vi "Update FLS Laser ID.vi"(8 "error in (no error)":errorcluster, 10 "DLS Laser ID (A,B,C or D)":enum16{"A", "B", "C", "D"}(ring), 11 "DLS Laser Actor in":refnum<class "FLS Laser Actor.lvclass">) -> (0 "error out":errorcluster, 3 "DLS Laser Actor out":refnum<class "FLS Laser Actor.lvclass">)   [LabVIEW 2018, in "FLS Laser Actor.lvlib" / "FLS Laser Actor.lvclass"]
uses:
  FLS Laser Actor.lvclass
  FLS Laser Actor.lvclass/FLS Laser Actor.ctl
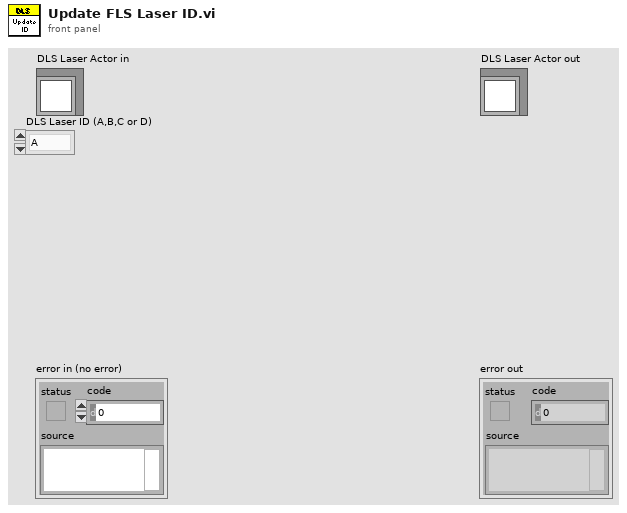
[diagram p1: front panel]
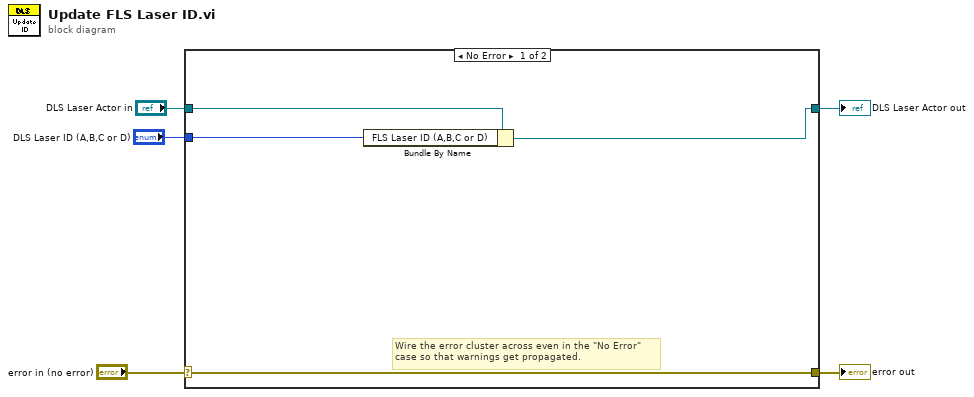
[diagram p0: block diagram]
diagram:
  n1 = case shown="No Error" "error in (no error)" {
    selector: "error in (no error)" -> [w9 w11]
    tunnel: [w9 w11] -> w4
    tunnel: [w7 w10] -> w2
    tunnel: "DLS Laser Actor in" -> [w8 w10]
    tunnel: "DLS Laser ID (A,B,C or D)" -> [w6 _]
    frame No Error {
      # "Wire the error cluster across even in the \"No Error\"\ncase so that warnings get propagated."
      n2 = Bundle By Name(cluster=w8, "FLS Laser ID (A,B,C or D)"=w6) -> (w7:refnum<class "FLS Laser Actor.lvclass">)
    }
    frame Error {
    }
  }
  "error out" <- w4
  "DLS Laser Actor out" <- w2
